vi "Find Device Config.vi"(8 "error in":errorcluster, 11 "Configuration in":refnum<class "Configuration.lvclass">) -> (0 "error out":errorcluster, 3 "Configuration out":refnum<class "Configuration.lvclass">)   [LabVIEW 2018, in "Configuration.lvlib" / "Configuration.lvclass"]
uses:
  Configuration.lvclass
  Configuration.lvclass/Configuration.ctl
  <vilib>/Utility/config.llb/Read Key (String).vi
  <vilib>/Utility/config.llb/NI_LVConfig.lvlib
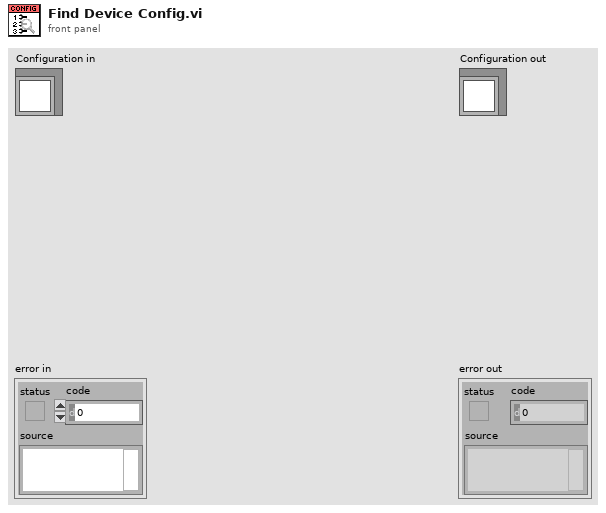
[diagram p1: front panel]
types:
  T1 = typedef "NI_LVConfig.lvlib/Config Data RefNum.ctl" = refnum<k1>
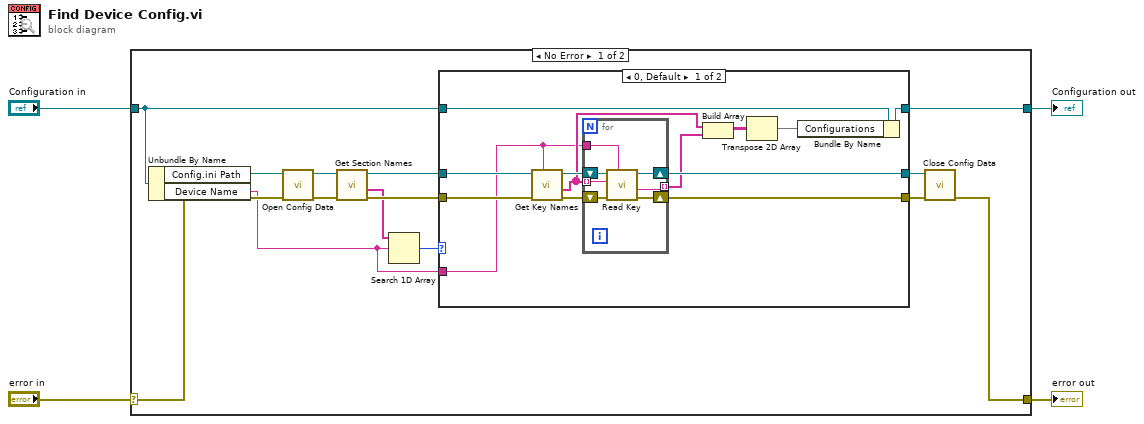
[diagram p0: block diagram]
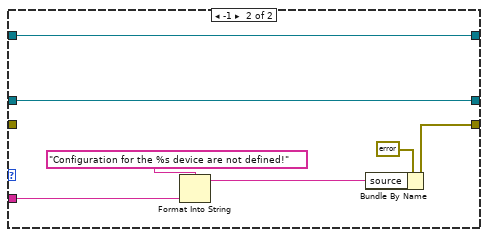
[diagram p2: hidden frame]
diagram:
  n1 = case shown="No Error" "error in" {
    selector: "error in" -> [w13 w47]
    tunnel: [w12 w47] -> w3
    tunnel: [w7 w46] -> w1
    tunnel: "Configuration in" -> [w8 w46]
    frame No Error {
      n2 = Unbundle By Name(w8) -> ("Config.ini Path"=w16:path, "Device Name"=w5:string)
      n3 = call <vilib>:"Open Config Data.vi"("error in (no error)"=w13, "configuration file path"=w16) -> ("error out"=w18:errorcluster, "refnum"=w17:T1)  [unwired: 7 in, 1 out]
      n4 = call <vilib>:"Get Section Names.vi"("error in (no error)"=w18, "refnum"=w17) -> ("error out"=w11:errorcluster, "section names"=w6:string[], "refnum out"=w15:T1)  [unwired: 7 in]
      n5 = Search 1D Array(1D array=w6, element=w5) -> (index of element=w9:i32)  [unwired: 1 in]
      n6 = case shown="0, Default" w9 {
        tunnel: w15 -> [w31 w45]
        tunnel: [w29 w45] -> w14
        tunnel: w11 -> [w28 _]
        tunnel: [w26 w42] -> w10
        tunnel: w8 -> [w23 w44]
        tunnel: [w21 w44] -> w7
        tunnel: w5 -> [w20 w39]
        frame 0, Default {
          n7 = call <vilib>:"Get Key Names.vi"("section"=w20, "error in (no error)"=w28, "refnum"=w31) -> ("error out"=w27:errorcluster, "key names"=w24:string[], "refnum out"=w30:T1)  [unwired: 5 in, 1 out]
          n8 = for {
            shift-right: [w37] -> w29
            shift-left: w30 -> [w38]
            shift-right: [w35] -> w26
            shift-left: w27 -> [w36]
            tunnel: w24 -> [w34] mode=indexing
            tunnel: [w33] -> w25 mode=indexing
            tunnel: w20 -> [w32]
            n9 = call-poly <vilib>:"Read Key.vi"("section"=w32, "error in (no error)"=w36, "key"=w34, "refnum"=w38) -> ("error out"=w35:errorcluster, "value"=w33:string, "refnum out"=w37:T1)  [unwired: 4 in, 1 out]
          }
          n10 = Build Array(w24, w25) -> (w22:string[][])
          n11 = Transpose 2D Array(2D array=w22) -> (transposed array=w19:string[][])
          n12 = Bundle By Name(cluster=w23, "Configurations"=w19) -> (w21:refnum<class "Configuration.lvclass">)
        }
        frame -1 {
          n13 = Format Into String(format string="Configuration for the %s device are not defined!", w39) -> (resulting string=w41:string)  [unwired: 2 in, 1 out]
          n14 = Bundle By Name(cluster=errorcluster {"status"=TRUE, "code"=-999, "source"=""} ("error out"), "source"=w41) -> (w42:errorcluster)
        }
      }
      n15 = call <vilib>:"Close Config Data.vi"("error in (no error)"=w10, "refnum"=w14) -> ("error out"=w12:errorcluster)  [unwired: 8 in, 1 out]
    }
    frame Error {
    }
  }
  "error out" <- w3
  "Configuration out" <- w1
